vi "S4GUI.vi"(7 "Tab ObsEng":enum32{"Obs", "CCD modes", "Eng"}(tab)) -> ()   [LabVIEW 2018] (continued)
            n3222 = call-dynamic "Write ObsType.vi"("error in (no error)"=w7236, "ObsType"=w7222, "Interface in"=w7230) -> ("error out"=w7235:errorcluster, "Interface out"=w7229:refnum<class "Interface.lvclass">)  [unwired: 7 in]
            n3223 = call-dynamic "Write Object.vi"("error in (no error)"=w7235, "Object"=w7221, "Interface in"=w7229) -> ("error out"=w7234:errorcluster, "Interface out"=w7228:refnum<class "Interface.lvclass">)  [unwired: 7 in]
            n3224 = call-dynamic "Write Comments.vi"("error in (no error)"=w7234, "Comments"=w7223, "Interface in"=w7228) -> ("error out"=w7215:errorcluster, "Interface out"=w7214:refnum<class "Interface.lvclass">)  [unwired: 7 in]
            n3225 = call-dynamic "Write Observer.vi"("error in (no error)"=w7215, "Observer"=w7220, "Interface in"=w7214) -> ("error out"=w7216:errorcluster, "Interface out"=w7217:refnum<class "Interface.lvclass">)  [unwired: 7 in]
            n3226 = call-dynamic "Write Interface.vi"("error in (no error)"=w7216, "Interface.lvclass"=w7217, "Channel in"=w7231) -> ("error out"=w7212:errorcluster, "Channel out"=w7213:refnum<class "Channel.lvclass">)  [unwired: 7 in]
            n3227 = disable-structure shown="Enabled" {
              disable-tunnel: w7213 -> [w7248 w7253]
              disable-tunnel: w7212 -> [w7247 w7252]
              disable-tunnel: [w7245 w7253] -> w7211
              disable-tunnel: [w7242 w7252] -> w7210
              frame Disabled {
                n3228 = call-dynamic "Read State Machine.vi"("error in (no error)"=w7247, "Device in"=w7248) -> ("error out"=w7251:errorcluster, "State Machine.lvclass"=w7244:refnum<class "State Machine.lvclass">, "Device out"=w7246:refnum<class "Channel.lvclass">)  [unwired: 7 in]
                n3229 = call "Next State.vi"("error in (no error)"=w7251, "New_State"=12, "State Machine in"=w7244) -> ("error out"=w7250:errorcluster, "State Machine out"=w7243:refnum<class "State Machine.lvclass">)  [unwired: 7 in]
                n3230 = call-dynamic "Write State Machine.vi"("error in (no error)"=w7250, "State Machine.lvclass"=w7243, "Device in"=w7246) -> ("error out"=w7242:errorcluster, "Device out"=w7245:refnum<class "Channel.lvclass">)  [unwired: 7 in]
              }
              frame Enabled {
              }
            }
            n3231 = call-dynamic "Write Channel.vi"("error in (no error)"=w7210, "Channel.lvclass"=w7211, "Acquisition in"=w7226) -> ("error out"=w7224:errorcluster, "Acquisition out"=w7225:refnum<class "Acquisition.lvclass">)  [unwired: 7 in]
            n3232 = call-dynamic "Write AcquisitionC.vi"("error in (no error)"=w7224, "Acquisition.lvclass"=w7225, "S4ACS_GUI in"=w7227) -> ("error out"=w7238:errorcluster, "S4ACS_GUI out"=w7239:refnum<class "S4GUI.lvclass">)  [unwired: 7 in]
          }
          frame #3 {
            # "object"
            # "suffix"
            # "obsType"
            n3233 = call-dynamic "Read AcquisitionD.vi"("error in (no error)"=w7289, "S4ACS_GUI in"=w7290) -> ("error out"=w7282:errorcluster, "Acquisition.lvclass"=w7281:refnum<class "Acquisition.lvclass">, "S4ACS_GUI out"=w7276:refnum<class "S4GUI.lvclass">)  [unwired: 7 in]
            n3234 = call-dynamic "Read Channel.vi"("error in (no error)"=w7282, "Acquisition in"=w7281) -> ("error out"=w7255:errorcluster, "Channel.lvclass"=w7257:refnum<class "Channel.lvclass">, "Acquisition out"=w7275:refnum<class "Acquisition.lvclass">)  [unwired: 7 in]
            n3235 = local read "Filter4"() -> (w7258:u8)
            n3236 = call-dynamic "Write Filter.vi"("error in (no error)"=w7255, "Filter"=w7258, "Channel in"=w7257) -> ("error out"=w7254:errorcluster, "Channel out"=w7256:refnum<class "Channel.lvclass">)  [unwired: 7 in]
            n3237 = call-dynamic "Read Interface.vi"("error in (no error)"=w7254, "Channel in"=w7256) -> ("error out"=w7267:errorcluster, "Interface.lvclass"=w7268:refnum<class "Interface.lvclass">, "Channel out"=w7280:refnum<class "Channel.lvclass">)  [unwired: 7 in]
            n3238 = call-dynamic "Write Suffix.vi"("error in (no error)"=w7267, "Suffix"=w7286, "Interface in"=w7268) -> ("error out"=w7285:errorcluster, "Interface out"=w7279:refnum<class "Interface.lvclass">)  [unwired: 7 in]
            n3239 = call-dynamic "Write ObsType.vi"("error in (no error)"=w7285, "ObsType"=w7271, "Interface in"=w7279) -> ("error out"=w7284:errorcluster, "Interface out"=w7278:refnum<class "Interface.lvclass">)  [unwired: 7 in]
            n3240 = call-dynamic "Write Object.vi"("error in (no error)"=w7284, "Object"=w7270, "Interface in"=w7278) -> ("error out"=w7283:errorcluster, "Interface out"=w7277:refnum<class "Interface.lvclass">)  [unwired: 7 in]
            n3241 = call-dynamic "Write Comments.vi"("error in (no error)"=w7283, "Comments"=w7272, "Interface in"=w7277) -> ("error out"=w7266:errorcluster, "Interface out"=w7265:refnum<class "Interface.lvclass">)  [unwired: 7 in]
            n3242 = call-dynamic "Write Observer.vi"("error in (no error)"=w7266, "Observer"=w7269, "Interface in"=w7265) -> ("error out"=w7264:errorcluster, "Interface out"=w7263:refnum<class "Interface.lvclass">)  [unwired: 7 in]
            n3243 = call-dynamic "Write Interface.vi"("error in (no error)"=w7264, "Interface.lvclass"=w7263, "Channel in"=w7280) -> ("error out"=w7260:errorcluster, "Channel out"=w7262:refnum<class "Channel.lvclass">)  [unwired: 7 in]
            n3244 = disable-structure shown="Enabled" {
              disable-tunnel: w7262 -> [w7297 w7302]
              disable-tunnel: [w7295 w7302] -> w7261
              disable-tunnel: w7260 -> [w7294 w7301]
              disable-tunnel: [w7293 w7301] -> w7259
              frame Disabled {
                n3245 = call-dynamic "Read State Machine.vi"("error in (no error)"=w7294, "Device in"=w7297) -> ("error out"=w7300:errorcluster, "State Machine.lvclass"=w7292:refnum<class "State Machine.lvclass">, "Device out"=w7296:refnum<class "Channel.lvclass">)  [unwired: 7 in]
                n3246 = call "Next State.vi"("error in (no error)"=w7300, "New_State"=12, "State Machine in"=w7292) -> ("error out"=w7299:errorcluster, "State Machine out"=w7291:refnum<class "State Machine.lvclass">)  [unwired: 7 in]
                n3247 = call-dynamic "Write State Machine.vi"("error in (no error)"=w7299, "State Machine.lvclass"=w7291, "Device in"=w7296) -> ("error out"=w7293:errorcluster, "Device out"=w7295:refnum<class "Channel.lvclass">)  [unwired: 7 in]
              }
              frame Enabled {
              }
            }
            n3248 = call-dynamic "Write Channel.vi"("error in (no error)"=w7259, "Channel.lvclass"=w7261, "Acquisition in"=w7275) -> ("error out"=w7273:errorcluster, "Acquisition out"=w7274:refnum<class "Acquisition.lvclass">)  [unwired: 7 in]
            n3249 = call-dynamic "Write AcquisitionD.vi"("error in (no error)"=w7273, "Acquisition.lvclass"=w7274, "S4ACS_GUI in"=w7276) -> ("error out"=w7287:errorcluster, "S4ACS_GUI out"=w7288:refnum<class "S4GUI.lvclass">)  [unwired: 7 in]
          }
        }
      }
      event "Observer": Value Change {
        n3250 = event-data() -> ("NewVal"=w7303:string)  [unwired: 1 in, 5 out]
        n3251 = disable-structure shown="Disabled" {
          disable-tunnel: w7306 -> [w7321 w7322]
          disable-tunnel: w7303 -> [w7320 _]
          disable-tunnel: [w7319 w7322] -> w7305
          frame Disabled {
            n3252 = String Length(string=w7320) -> (length=w7318:i32)
            n3253 = Equal To 0?(x=w7318) -> (x = 0?=w7317:bool)
            n3254 = Select(t=u32 16777216, s=w7317, f=u32 16777225) -> (s? t:f=w7315:u32)
            n3255 = property on="Observer" class="Str"(error in=w7321, "Text.BGColor"=w7315) -> (error out=w7319:errorcluster)  [unwired: 1 in, 1 out]
          }
          frame Enabled {
            # "Não se usa mais o texto de fundo\ndo controle \"Observer\""
          }
        }
        n3256 = case shown="False" FALSE {
          tunnel: w7313 -> [w7331 w7529]
          tunnel: w7312 -> [w7330 _]
          tunnel: w7311 -> [w7329 _]
          tunnel: w7310 -> [w7328 _]
          tunnel: w7303 -> [w7327 _]
          tunnel: w7309 -> [w7326 _]
          tunnel: [w7325 w7529] -> w7308
          tunnel: [w7324 w7528] -> w7307
          tunnel: w7305 -> [w7323 w7528]
          frame False {
            n3257 = stacked-sequence {
              seq-local: [w7353 _ _ _] -> [_ w7417 _ _]
              seq-local: [w7352 _ _ _] -> [_ w7416 _ _]
              seq-local: [_ w7415 _ _] -> [_ _ w7466 _]
              seq-local: [_ w7414 _ _] -> [_ _ w7465 _]
              seq-local: [_ _ w7464 _] -> [_ _ _ w7515]
              seq-local: [_ _ w7463 _] -> [_ _ _ w7514]
              tunnel: w7323 -> [w7365 _ _ _]
              tunnel: w7331 -> [w7364 _ _ _]
              tunnel: [_ _ _ w7513] -> w7325
              tunnel: [_ _ _ w7512] -> w7324
              tunnel: w7329 -> [w7351 w7413 w7462 w7511]
              tunnel: w7328 -> [w7350 w7412 w7448 w7497]
              tunnel: w7326 -> [w7349 w7398 w7447 w7496]
              tunnel: w7330 -> [w7348 w7397 w7446 w7495]
              tunnel: w7327 -> [w7347 w7396 w7445 w7494]
              frame #0 {
                # "observer"
                # "comment"
                # "object"
                # "suffix"
                # "obsType"
                n3258 = call-dynamic "Read AcquisitionA.vi"("error in (no error)"=w7365, "S4ACS_GUI in"=w7364) -> ("error out"=w7363:errorcluster, "Acquisition.lvclass"=w7362:refnum<class "Acquisition.lvclass">, "S4ACS_GUI out"=w7357:refnum<class "S4GUI.lvclass">)  [unwired: 7 in]
                n3259 = call-dynamic "Read Channel.vi"("error in (no error)"=w7363, "Acquisition in"=w7362) -> ("error out"=w7333:errorcluster, "Channel.lvclass"=w7336:refnum<class "Channel.lvclass">, "Acquisition out"=w7356:refnum<class "Acquisition.lvclass">)  [unwired: 7 in]
                n3260 = local read "Filter1"() -> (w7334:u8)
                n3261 = call-dynamic "Write Filter.vi"("error in (no error)"=w7333, "Filter"=w7334, "Channel in"=w7336) -> ("error out"=w7332:errorcluster, "Channel out"=w7335:refnum<class "Channel.lvclass">)  [unwired: 7 in]
                n3262 = call-dynamic "Read Interface.vi"("error in (no error)"=w7332, "Channel in"=w7335) -> ("error out"=w7343:errorcluster, "Interface.lvclass"=w7344:refnum<class "Interface.lvclass">, "Channel out"=w7361:refnum<class "Channel.lvclass">)  [unwired: 7 in]
                n3263 = call-dynamic "Write Suffix.vi"("error in (no error)"=w7343, "Suffix"=w7351, "Interface in"=w7344) -> ("error out"=w7368:errorcluster, "Interface out"=w7360:refnum<class "Interface.lvclass">)  [unwired: 7 in]
                n3264 = call-dynamic "Write ObsType.vi"("error in (no error)"=w7368, "ObsType"=w7349, "Interface in"=w7360) -> ("error out"=w7367:errorcluster, "Interface out"=w7359:refnum<class "Interface.lvclass">)  [unwired: 7 in]
                n3265 = call-dynamic "Write Object.vi"("error in (no error)"=w7367, "Object"=w7348, "Interface in"=w7359) -> ("error out"=w7366:errorcluster, "Interface out"=w7358:refnum<class "Interface.lvclass">)  [unwired: 7 in]
                n3266 = call-dynamic "Write Comments.vi"("error in (no error)"=w7366, "Comments"=w7350, "Interface in"=w7358) -> ("error out"=w7346:errorcluster, "Interface out"=w7345:refnum<class "Interface.lvclass">)  [unwired: 7 in]
                n3267 = call-dynamic "Write Observer.vi"("error in (no error)"=w7346, "Observer"=w7347, "Interface in"=w7345) -> ("error out"=w7341:errorcluster, "Interface out"=w7342:refnum<class "Interface.lvclass">)  [unwired: 7 in]
                n3268 = call-dynamic "Write Interface.vi"("error in (no error)"=w7341, "Interface.lvclass"=w7342, "Channel in"=w7361) -> ("error out"=w7338:errorcluster, "Channel out"=w7340:refnum<class "Channel.lvclass">)  [unwired: 7 in]
                n3269 = disable-structure shown="Enabled" {
                  disable-tunnel: w7340 -> [w7378 w7380]
                  disable-tunnel: [w7376 w7380] -> w7339
                  disable-tunnel: w7338 -> [w7375 w7379]
                  disable-tunnel: [w7370 w7379] -> w7337
                  frame Disabled {
                    n3270 = call-dynamic "Read State Machine.vi"("error in (no error)"=w7375, "Device in"=w7378) -> ("error out"=w7374:errorcluster, "State Machine.lvclass"=w7372:refnum<class "State Machine.lvclass">, "Device out"=w7377:refnum<class "Channel.lvclass">)  [unwired: 7 in]
                    n3271 = call "Next State.vi"("error in (no error)"=w7374, "New_State"=12, "State Machine in"=w7372) -> ("error out"=w7373:errorcluster, "State Machine out"=w7371:refnum<class "State Machine.lvclass">)  [unwired: 7 in]
                    n3272 = call-dynamic "Write State Machine.vi"("error in (no error)"=w7373, "State Machine.lvclass"=w7371, "Device in"=w7377) -> ("error out"=w7370:errorcluster, "Device out"=w7376:refnum<class "Channel.lvclass">)  [unwired: 7 in]
                  }
                  frame Enabled {
                  }
                }
                n3273 = call-dynamic "Write Channel.vi"("error in (no error)"=w7337, "Channel.lvclass"=w7339, "Acquisition in"=w7356) -> ("error out"=w7354:errorcluster, "Acquisition out"=w7355:refnum<class "Acquisition.lvclass">)  [unwired: 7 in]
                n3274 = call-dynamic "Write AcquisitionA.vi"("error in (no error)"=w7354, "Acquisition.lvclass"=w7355, "S4ACS_GUI in"=w7357) -> ("error out"=w7352:errorcluster, "S4ACS_GUI out"=w7353:refnum<class "S4GUI.lvclass">)  [unwired: 7 in]
              }
              frame #1 {
                # "object"
                # "suffix"
                # "obsType"
                n3275 = call "Read AcquisitionB.vi"("error in (no error)"=w7416, "S4ACS_GUI in"=w7417) -> ("error out"=w7402:errorcluster, "Acquisition.lvclass"=w7403:refnum<class "Acquisition.lvclass">, "S4ACS_GUI out"=w7408:refnum<class "S4GUI.lvclass">)  [unwired: 7 in]
                n3276 = call-dynamic "Read Channel.vi"("error in (no error)"=w7402, "Acquisition in"=w7403) -> ("error out"=w7382:errorcluster, "Channel.lvclass"=w7384:refnum<class "Channel.lvclass">, "Acquisition out"=w7409:refnum<class "Acquisition.lvclass">)  [unwired: 7 in]
                n3277 = local read "Filter2"() -> (w7385:u8)
                n3278 = call-dynamic "Write Filter.vi"("error in (no error)"=w7382, "Filter"=w7385, "Channel in"=w7384) -> ("error out"=w7381:errorcluster, "Channel out"=w7383:refnum<class "Channel.lvclass">)  [unwired: 7 in]
                n3279 = call-dynamic "Read Interface.vi"("error in (no error)"=w7381, "Channel in"=w7383) -> ("error out"=w7390:errorcluster, "Interface.lvclass"=w7391:refnum<class "Interface.lvclass">, "Channel out"=w7404:refnum<class "Channel.lvclass">)  [unwired: 7 in]
                n3280 = call-dynamic "Write Suffix.vi"("error in (no error)"=w7390, "Suffix"=w7413, "Interface in"=w7391) -> ("error out"=w7399:errorcluster, "Interface out"=w7405:refnum<class "Interface.lvclass">)  [unwired: 7 in]
                n3281 = call-dynamic "Write ObsType.vi"("error in (no error)"=w7399, "ObsType"=w7398, "Interface in"=w7405) -> ("error out"=w7400:errorcluster, "Interface out"=w7406:refnum<class "Interface.lvclass">)  [unwired: 7 in]
                n3282 = call-dynamic "Write Object.vi"("error in (no error)"=w7400, "Object"=w7397, "Interface in"=w7406) -> ("error out"=w7401:errorcluster, "Interface out"=w7407:refnum<class "Interface.lvclass">)  [unwired: 7 in]
                n3283 = call-dynamic "Write Comments.vi"("error in (no error)"=w7401, "Comments"=w7412, "Interface in"=w7407) -> ("error out"=w7393:errorcluster, "Interface out"=w7392:refnum<class "Interface.lvclass">)  [unwired: 7 in]
                n3284 = call-dynamic "Write Observer.vi"("error in (no error)"=w7393, "Observer"=w7396, "Interface in"=w7392) -> ("error out"=w7394:errorcluster, "Interface out"=w7395:refnum<class "Interface.lvclass">)  [unwired: 7 in]
                n3285 = call-dynamic "Write Interface.vi"("error in (no error)"=w7394, "Interface.lvclass"=w7395, "Channel in"=w7404) -> ("error out"=w7388:errorcluster, "Channel out"=w7389:refnum<class "Channel.lvclass">)  [unwired: 7 in]
                n3286 = disable-structure shown="Enabled" {
                  disable-tunnel: w7389 -> [w7422 w7429]
                  disable-tunnel: w7388 -> [w7421 w7428]
                  disable-tunnel: [w7419 w7429] -> w7387
                  disable-tunnel: [w7418 w7428] -> w7386
                  frame Disabled {
                    n3287 = call-dynamic "Read State Machine.vi"("error in (no error)"=w7421, "Device in"=w7422) -> ("error out"=w7427:errorcluster, "State Machine.lvclass"=w7425:refnum<class "State Machine.lvclass">, "Device out"=w7420:refnum<class "Channel.lvclass">)  [unwired: 7 in]
                    n3288 = call "Next State.vi"("error in (no error)"=w7427, "New_State"=12, "State Machine in"=w7425) -> ("error out"=w7426:errorcluster, "State Machine out"=w7424:refnum<class "State Machine.lvclass">)  [unwired: 7 in]
                    n3289 = call-dynamic "Write State Machine.vi"("error in (no error)"=w7426, "State Machine.lvclass"=w7424, "Device in"=w7420) -> ("error out"=w7418:errorcluster, "Device out"=w7419:refnum<class "Channel.lvclass">)  [unwired: 7 in]
                  }
                  frame Enabled {
                  }
                }
                n3290 = call-dynamic "Write Channel.vi"("error in (no error)"=w7386, "Channel.lvclass"=w7387, "Acquisition in"=w7409) -> ("error out"=w7411:errorcluster, "Acquisition out"=w7410:refnum<class "Acquisition.lvclass">)  [unwired: 7 in]
                n3291 = call "Write AcquisitionB.vi"("error in (no error)"=w7411, "Acquisition.lvclass"=w7410, "S4ACS_GUI in"=w7408) -> ("error out"=w7414:errorcluster, "S4ACS_GUI out"=w7415:refnum<class "S4GUI.lvclass">)  [unwired: 7 in]
              }
              frame #2 {
                # "object"
                # "suffix"
                # "obsType"
                n3292 = call-dynamic "Read AcquisitionC.vi"("error in (no error)"=w7465, "S4ACS_GUI in"=w7466) -> ("error out"=w7458:errorcluster, "Acquisition.lvclass"=w7457:refnum<class "Acquisition.lvclass">, "S4ACS_GUI out"=w7452:refnum<class "S4GUI.lvclass">)  [unwired: 7 in]
                n3293 = call-dynamic "Read Channel.vi"("error in (no error)"=w7458, "Acquisition in"=w7457) -> ("error out"=w7431:errorcluster, "Channel.lvclass"=w7433:refnum<class "Channel.lvclass">, "Acquisition out"=w7451:refnum<class "Acquisition.lvclass">)  [unwired: 7 in]
                n3294 = local read "Filter3"() -> (w7434:u8)
                n3295 = call-dynamic "Write Filter.vi"("error in (no error)"=w7431, "Filter"=w7434, "Channel in"=w7433) -> ("error out"=w7430:errorcluster, "Channel out"=w7432:refnum<class "Channel.lvclass">)  [unwired: 7 in]
                n3296 = call-dynamic "Read Interface.vi"("error in (no error)"=w7430, "Channel in"=w7432) -> ("error out"=w7443:errorcluster, "Interface.lvclass"=w7444:refnum<class "Interface.lvclass">, "Channel out"=w7456:refnum<class "Channel.lvclass">)  [unwired: 7 in]
                n3297 = call-dynamic "Write Suffix.vi"("error in (no error)"=w7443, "Suffix"=w7462, "Interface in"=w7444) -> ("error out"=w7461:errorcluster, "Interface out"=w7455:refnum<class "Interface.lvclass">)  [unwired: 7 in]
                n3298 = call-dynamic "Write ObsType.vi"("error in (no error)"=w7461, "ObsType"=w7447, "Interface in"=w7455) -> ("error out"=w7460:errorcluster, "Interface out"=w7454:refnum<class "Interface.lvclass">)  [unwired: 7 in]
                n3299 = call-dynamic "Write Object.vi"("error in (no error)"=w7460, "Object"=w7446, "Interface in"=w7454) -> ("error out"=w7459:errorcluster, "Interface out"=w7453:refnum<class "Interface.lvclass">)  [unwired: 7 in]
                n3300 = call-dynamic "Write Comments.vi"("error in (no error)"=w7459, "Comments"=w7448, "Interface in"=w7453) -> ("error out"=w7440:errorcluster, "Interface out"=w7439:refnum<class "Interface.lvclass">)  [unwired: 7 in]
                n3301 = call-dynamic "Write Observer.vi"("error in (no error)"=w7440, "Observer"=w7445, "Interface in"=w7439) -> ("error out"=w7441:errorcluster, "Interface out"=w7442:refnum<class "Interface.lvclass">)  [unwired: 7 in]
                n3302 = call-dynamic "Write Interface.vi"("error in (no error)"=w7441, "Interface.lvclass"=w7442, "Channel in"=w7456) -> ("error out"=w7437:errorcluster, "Channel out"=w7438:refnum<class "Channel.lvclass">)  [unwired: 7 in]
                n3303 = disable-structure shown="Enabled" {
                  disable-tunnel: w7438 -> [w7473 w7478]
                  disable-tunnel: w7437 -> [w7472 w7477]
                  disable-tunnel: [w7470 w7478] -> w7436
                  disable-tunnel: [w7467 w7477] -> w7435
                  frame Disabled {
                    n3304 = call-dynamic "Read State Machine.vi"("error in (no error)"=w7472, "Device in"=w7473) -> ("error out"=w7476:errorcluster, "State Machine.lvclass"=w7469:refnum<class "State Machine.lvclass">, "Device out"=w7471:refnum<class "Channel.lvclass">)  [unwired: 7 in]
                    n3305 = call "Next State.vi"("error in (no error)"=w7476, "New_State"=12, "State Machine in"=w7469) -> ("error out"=w7475:errorcluster, "State Machine out"=w7468:refnum<class "State Machine.lvclass">)  [unwired: 7 in]
                    n3306 = call-dynamic "Write State Machine.vi"("error in (no error)"=w7475, "State Machine.lvclass"=w7468, "Device in"=w7471) -> ("error out"=w7467:errorcluster, "Device out"=w7470:refnum<class "Channel.lvclass">)  [unwired: 7 in]
                  }
                  frame Enabled {
                  }
                }
                n3307 = call-dynamic "Write Channel.vi"("error in (no error)"=w7435, "Channel.lvclass"=w7436, "Acquisition in"=w7451) -> ("error out"=w7449:errorcluster, "Acquisition out"=w7450:refnum<class "Acquisition.lvclass">)  [unwired: 7 in]
                n3308 = call-dynamic "Write AcquisitionC.vi"("error in (no error)"=w7449, "Acquisition.lvclass"=w7450, "S4ACS_GUI in"=w7452) -> ("error out"=w7463:errorcluster, "S4ACS_GUI out"=w7464:refnum<class "S4GUI.lvclass">)  [unwired: 7 in]
              }
              frame #3 {
                # "object"
                # "suffix"
                # "obsType"
                n3309 = call-dynamic "Read AcquisitionD.vi"("error in (no error)"=w7514, "S4ACS_GUI in"=w7515) -> ("error out"=w7507:errorcluster, "Acquisition.lvclass"=w7506:refnum<class "Acquisition.lvclass">, "S4ACS_GUI out"=w7501:refnum<class "S4GUI.lvclass">)  [unwired: 7 in]
                n3310 = call-dynamic "Read Channel.vi"("error in (no error)"=w7507, "Acquisition in"=w7506) -> ("error out"=w7480:errorcluster, "Channel.lvclass"=w7482:refnum<class "Channel.lvclass">, "Acquisition out"=w7500:refnum<class "Acquisition.lvclass">)  [unwired: 7 in]
                n3311 = local read "Filter4"() -> (w7483:u8)
                n3312 = call-dynamic "Write Filter.vi"("error in (no error)"=w7480, "Filter"=w7483, "Channel in"=w7482) -> ("error out"=w7479:errorcluster, "Channel out"=w7481:refnum<class "Channel.lvclass">)  [unwired: 7 in]
                n3313 = call-dynamic "Read Interface.vi"("error in (no error)"=w7479, "Channel in"=w7481) -> ("error out"=w7492:errorcluster, "Interface.lvclass"=w7493:refnum<class "Interface.lvclass">, "Channel out"=w7505:refnum<class "Channel.lvclass">)  [unwired: 7 in]
                n3314 = call-dynamic "Write Suffix.vi"("error in (no error)"=w7492, "Suffix"=w7511, "Interface in"=w7493) -> ("error out"=w7510:errorcluster, "Interface out"=w7504:refnum<class "Interface.lvclass">)  [unwired: 7 in]
                n3315 = call-dynamic "Write ObsType.vi"("error in (no error)"=w7510, "ObsType"=w7496, "Interface in"=w7504) -> ("error out"=w7509:errorcluster, "Interface out"=w7503:refnum<class "Interface.lvclass">)  [unwired: 7 in]
                n3316 = call-dynamic "Write Object.vi"("error in (no error)"=w7509, "Object"=w7495, "Interface in"=w7503) -> ("error out"=w7508:errorcluster, "Interface out"=w7502:refnum<class "Interface.lvclass">)  [unwired: 7 in]
                n3317 = call-dynamic "Write Comments.vi"("error in (no error)"=w7508, "Comments"=w7497, "Interface in"=w7502) -> ("error out"=w7491:errorcluster, "Interface out"=w7490:refnum<class "Interface.lvclass">)  [unwired: 7 in]
                n3318 = call-dynamic "Write Observer.vi"("error in (no error)"=w7491, "Observer"=w7494, "Interface in"=w7490) -> ("error out"=w7489:errorcluster, "Interface out"=w7488:refnum<class "Interface.lvclass">)  [unwired: 7 in]
                n3319 = call-dynamic "Write Interface.vi"("error in (no error)"=w7489, "Interface.lvclass"=w7488, "Channel in"=w7505) -> ("error out"=w7485:errorcluster, "Channel out"=w7487:refnum<class "Channel.lvclass">)  [unwired: 7 in]
                n3320 = disable-structure shown="Enabled" {
                  disable-tunnel: w7487 -> [w7522 w7527]
                  disable-tunnel: [w7520 w7527] -> w7486
                  disable-tunnel: w7485 -> [w7519 w7526]
                  disable-tunnel: [w7518 w7526] -> w7484
                  frame Disabled {
                    n3321 = call-dynamic "Read State Machine.vi"("error in (no error)"=w7519, "Device in"=w7522) -> ("error out"=w7525:errorcluster, "State Machine.lvclass"=w7517:refnum<class "State Machine.lvclass">, "Device out"=w7521:refnum<class "Channel.lvclass">)  [unwired: 7 in]
                    n3322 = call "Next State.vi"("error in (no error)"=w7525, "New_State"=12, "State Machine in"=w7517) -> ("error out"=w7524:errorcluster, "State Machine out"=w7516:refnum<class "State Machine.lvclass">)  [unwired: 7 in]
                    n3323 = call-dynamic "Write State Machine.vi"("error in (no error)"=w7524, "State Machine.lvclass"=w7516, "Device in"=w7521) -> ("error out"=w7518:errorcluster, "Device out"=w7520:refnum<class "Channel.lvclass">)  [unwired: 7 in]
                  }
                  frame Enabled {
                  }
                }
                n3324 = call-dynamic "Write Channel.vi"("error in (no error)"=w7484, "Channel.lvclass"=w7486, "Acquisition in"=w7500) -> ("error out"=w7498:errorcluster, "Acquisition out"=w7499:refnum<class "Acquisition.lvclass">)  [unwired: 7 in]
                n3325 = call-dynamic "Write AcquisitionD.vi"("error in (no error)"=w7498, "Acquisition.lvclass"=w7499, "S4ACS_GUI in"=w7501) -> ("error out"=w7512:errorcluster, "S4ACS_GUI out"=w7513:refnum<class "S4GUI.lvclass">)  [unwired: 7 in]
              }
            }
          }
          frame True {
          }
        }
      }
      event "Observer": Mouse Enter {
        n3326 = event-data() -> ()  [unwired: 1 in, 4 out]
        n3327 = disable-structure shown="Disabled" {
          disable-tunnel: [w7535 w7538] -> w7531
          disable-tunnel: w7530 -> [w7533 w7538]
          frame Disabled {
            n3328 = property on="Observer" class="Str"() -> ("Value"=w7534:string)  [unwired: 2 in, 2 out]
            n3329 = String Length(string=w7534) -> (length=w7537:i32)
            n3330 = Equal To 0?(x=w7537) -> (x = 0?=w7536:bool)
            n3331 = property on="Observer" class="Str"(error in=w7533, "Caption.Visible"=w7536) -> (error out=w7535:errorcluster)  [unwired: 1 in, 1 out]
          }
          frame Enabled {
            # "Não se usa mais o texto de fundo\ndo controle \"Observer\""
          }
        }
      }
      event "Filter1", "Filter2", "Filter3", "Filter4": Value Change {
        n3332 = event-data() -> ()  [unwired: 1 in, 6 out]
        n3333 = stacked-sequence {
          seq-local: [w7569 _ _ _] -> [_ w7633 _ _]
          seq-local: [w7568 _ _ _] -> [_ w7632 _ _]
          seq-local: [_ w7631 _ _] -> [_ _ w7682 _]
          seq-local: [_ w7630 _ _] -> [_ _ w7681 _]
          seq-local: [_ _ w7680 _] -> [_ _ _ w7731]
          seq-local: [_ _ w7679 _] -> [_ _ _ w7730]
          tunnel: w7546 -> [w7581 _ _ _]
          tunnel: w7547 -> [w7580 _ _ _]
          tunnel: [_ _ _ w7729] -> w7540
          tunnel: [_ _ _ w7728] -> w7539
          tunnel: w7544 -> [w7567 w7629 w7678 w7727]
          tunnel: w7543 -> [w7566 w7628 w7664 w7713]
          tunnel: w7541 -> [w7565 w7614 w7663 w7712]
          tunnel: w7545 -> [w7564 w7613 w7662 w7711]
          tunnel: w7542 -> [w7563 w7612 w7661 w7710]
          frame #0 {
            # "observer"
            # "comment"
            # "object"
            # "suffix"
            # "obsType"
            n3334 = call-dynamic "Read AcquisitionA.vi"("error in (no error)"=w7581, "S4ACS_GUI in"=w7580) -> ("error out"=w7579:errorcluster, "Acquisition.lvclass"=w7578:refnum<class "Acquisition.lvclass">, "S4ACS_GUI out"=w7573:refnum<class "S4GUI.lvclass">)  [unwired: 7 in]
            n3335 = call-dynamic "Read Channel.vi"("error in (no error)"=w7579, "Acquisition in"=w7578) -> ("error out"=w7549:errorcluster, "Channel.lvclass"=w7552:refnum<class "Channel.lvclass">, "Acquisition out"=w7572:refnum<class "Acquisition.lvclass">)  [unwired: 7 in]
            n3336 = local read "Filter1"() -> (w7550:u8)
            n3337 = call-dynamic "Write Filter.vi"("error in (no error)"=w7549, "Filter"=w7550, "Channel in"=w7552) -> ("error out"=w7548:errorcluster, "Channel out"=w7551:refnum<class "Channel.lvclass">)  [unwired: 7 in]
            n3338 = call-dynamic "Read Interface.vi"("error in (no error)"=w7548, "Channel in"=w7551) -> ("error out"=w7559:errorcluster, "Interface.lvclass"=w7560:refnum<class "Interface.lvclass">, "Channel out"=w7577:refnum<class "Channel.lvclass">)  [unwired: 7 in]
            n3339 = call-dynamic "Write Suffix.vi"("error in (no error)"=w7559, "Suffix"=w7567, "Interface in"=w7560) -> ("error out"=w7584:errorcluster, "Interface out"=w7576:refnum<class "Interface.lvclass">)  [unwired: 7 in]
            n3340 = call-dynamic "Write ObsType.vi"("error in (no error)"=w7584, "ObsType"=w7565, "Interface in"=w7576) -> ("error out"=w7583:errorcluster, "Interface out"=w7575:refnum<class "Interface.lvclass">)  [unwired: 7 in]
            n3341 = call-dynamic "Write Object.vi"("error in (no error)"=w7583, "Object"=w7564, "Interface in"=w7575) -> ("error out"=w7582:errorcluster, "Interface out"=w7574:refnum<class "Interface.lvclass">)  [unwired: 7 in]
            n3342 = call-dynamic "Write Comments.vi"("error in (no error)"=w7582, "Comments"=w7566, "Interface in"=w7574) -> ("error out"=w7562:errorcluster, "Interface out"=w7561:refnum<class "Interface.lvclass">)  [unwired: 7 in]
            n3343 = call-dynamic "Write Observer.vi"("error in (no error)"=w7562, "Observer"=w7563, "Interface in"=w7561) -> ("error out"=w7557:errorcluster, "Interface out"=w7558:refnum<class "Interface.lvclass">)  [unwired: 7 in]
            n3344 = call-dynamic "Write Interface.vi"("error in (no error)"=w7557, "Interface.lvclass"=w7558, "Channel in"=w7577) -> ("error out"=w7554:errorcluster, "Channel out"=w7556:refnum<class "Channel.lvclass">)  [unwired: 7 in]
            n3345 = disable-structure shown="Enabled" {
              disable-tunnel: w7556 -> [w7594 w7596]
              disable-tunnel: [w7592 w7596] -> w7555
              disable-tunnel: w7554 -> [w7591 w7595]
              disable-tunnel: [w7586 w7595] -> w7553
              frame Disabled {
                n3346 = call-dynamic "Read State Machine.vi"("error in (no error)"=w7591, "Device in"=w7594) -> ("error out"=w7590:errorcluster, "State Machine.lvclass"=w7588:refnum<class "State Machine.lvclass">, "Device out"=w7593:refnum<class "Channel.lvclass">)  [unwired: 7 in]
                n3347 = call "Next State.vi"("error in (no error)"=w7590, "New_State"=12, "State Machine in"=w7588) -> ("error out"=w7589:errorcluster, "State Machine out"=w7587:refnum<class "State Machine.lvclass">)  [unwired: 7 in]
                n3348 = call-dynamic "Write State Machine.vi"("error in (no error)"=w7589, "State Machine.lvclass"=w7587, "Device in"=w7593) -> ("error out"=w7586:errorcluster, "Device out"=w7592:refnum<class "Channel.lvclass">)  [unwired: 7 in]
              }
              frame Enabled {
              }
            }
            n3349 = call-dynamic "Write Channel.vi"("error in (no error)"=w7553, "Channel.lvclass"=w7555, "Acquisition in"=w7572) -> ("error out"=w7570:errorcluster, "Acquisition out"=w7571:refnum<class "Acquisition.lvclass">)  [unwired: 7 in]
            n3350 = call-dynamic "Write AcquisitionA.vi"("error in (no error)"=w7570, "Acquisition.lvclass"=w7571, "S4ACS_GUI in"=w7573) -> ("error out"=w7568:errorcluster, "S4ACS_GUI out"=w7569:refnum<class "S4GUI.lvclass">)  [unwired: 7 in]
          }
          frame #1 {
            # "object"
            # "suffix"
            # "obsType"
            n3351 = call "Read AcquisitionB.vi"("error in (no error)"=w7632, "S4ACS_GUI in"=w7633) -> ("error out"=w7618:errorcluster, "Acquisition.lvclass"=w7619:refnum<class "Acquisition.lvclass">, "S4ACS_GUI out"=w7624:refnum<class "S4GUI.lvclass">)  [unwired: 7 in]
            n3352 = call-dynamic "Read Channel.vi"("error in (no error)"=w7618, "Acquisition in"=w7619) -> ("error out"=w7598:errorcluster, "Channel.lvclass"=w7600:refnum<class "Channel.lvclass">, "Acquisition out"=w7625:refnum<class "Acquisition.lvclass">)  [unwired: 7 in]
            n3353 = local read "Filter2"() -> (w7601:u8)
            n3354 = call-dynamic "Write Filter.vi"("error in (no error)"=w7598, "Filter"=w7601, "Channel in"=w7600) -> ("error out"=w7597:errorcluster, "Channel out"=w7599:refnum<class "Channel.lvclass">)  [unwired: 7 in]
            n3355 = call-dynamic "Read Interface.vi"("error in (no error)"=w7597, "Channel in"=w7599) -> ("error out"=w7606:errorcluster, "Interface.lvclass"=w7607:refnum<class "Interface.lvclass">, "Channel out"=w7620:refnum<class "Channel.lvclass">)  [unwired: 7 in]
            n3356 = call-dynamic "Write Suffix.vi"("error in (no error)"=w7606, "Suffix"=w7629, "Interface in"=w7607) -> ("error out"=w7615:errorcluster, "Interface out"=w7621:refnum<class "Interface.lvclass">)  [unwired: 7 in]
            n3357 = call-dynamic "Write ObsType.vi"("error in (no error)"=w7615, "ObsType"=w7614, "Interface in"=w7621) -> ("error out"=w7616:errorcluster, "Interface out"=w7622:refnum<class "Interface.lvclass">)  [unwired: 7 in]
            n3358 = call-dynamic "Write Object.vi"("error in (no error)"=w7616, "Object"=w7613, "Interface in"=w7622) -> ("error out"=w7617:errorcluster, "Interface out"=w7623:refnum<class "Interface.lvclass">)  [unwired: 7 in]
            n3359 = call-dynamic "Write Comments.vi"("error in (no error)"=w7617, "Comments"=w7628, "Interface in"=w7623) -> ("error out"=w7609:errorcluster, "Interface out"=w7608:refnum<class "Interface.lvclass">)  [unwired: 7 in]
            n3360 = call-dynamic "Write Observer.vi"("error in (no error)"=w7609, "Observer"=w7612, "Interface in"=w7608) -> ("error out"=w7610:errorcluster, "Interface out"=w7611:refnum<class "Interface.lvclass">)  [unwired: 7 in]
            n3361 = call-dynamic "Write Interface.vi"("error in (no error)"=w7610, "Interface.lvclass"=w7611, "Channel in"=w7620) -> ("error out"=w7604:errorcluster, "Channel out"=w7605:refnum<class "Channel.lvclass">)  [unwired: 7 in]
            n3362 = disable-structure shown="Enabled" {
              disable-tunnel: w7605 -> [w7638 w7645]
              disable-tunnel: w7604 -> [w7637 w7644]
              disable-tunnel: [w7635 w7645] -> w7603
              disable-tunnel: [w7634 w7644] -> w7602
              frame Disabled {
                n3363 = call-dynamic "Read State Machine.vi"("error in (no error)"=w7637, "Device in"=w7638) -> ("error out"=w7643:errorcluster, "State Machine.lvclass"=w7641:refnum<class "State Machine.lvclass">, "Device out"=w7636:refnum<class "Channel.lvclass">)  [unwired: 7 in]
                n3364 = call "Next State.vi"("error in (no error)"=w7643, "New_State"=12, "State Machine in"=w7641) -> ("error out"=w7642:errorcluster, "State Machine out"=w7640:refnum<class "State Machine.lvclass">)  [unwired: 7 in]
                n3365 = call-dynamic "Write State Machine.vi"("error in (no error)"=w7642, "State Machine.lvclass"=w7640, "Device in"=w7636) -> ("error out"=w7634:errorcluster, "Device out"=w7635:refnum<class "Channel.lvclass">)  [unwired: 7 in]
              }
              frame Enabled {
              }
            }
            n3366 = call-dynamic "Write Channel.vi"("error in (no error)"=w7602, "Channel.lvclass"=w7603, "Acquisition in"=w7625) -> ("error out"=w7627:errorcluster, "Acquisition out"=w7626:refnum<class "Acquisition.lvclass">)  [unwired: 7 in]
            n3367 = call "Write AcquisitionB.vi"("error in (no error)"=w7627, "Acquisition.lvclass"=w7626, "S4ACS_GUI in"=w7624) -> ("error out"=w7630:errorcluster, "S4ACS_GUI out"=w7631:refnum<class "S4GUI.lvclass">)  [unwired: 7 in]
          }
          frame #2 {
            # "object"
            # "suffix"
            # "obsType"
            n3368 = call-dynamic "Read AcquisitionC.vi"("error in (no error)"=w7681, "S4ACS_GUI in"=w7682) -> ("error out"=w7674:errorcluster, "Acquisition.lvclass"=w7673:refnum<class "Acquisition.lvclass">, "S4ACS_GUI out"=w7668:refnum<class "S4GUI.lvclass">)  [unwired: 7 in]
            n3369 = call-dynamic "Read Channel.vi"("error in (no error)"=w7674, "Acquisition in"=w7673) -> ("error out"=w7648:errorcluster, "Channel.lvclass"=w7650:refnum<class "Channel.lvclass">, "Acquisition out"=w7667:refnum<class "Acquisition.lvclass">)  [unwired: 7 in]
            n3370 = local read "Filter3"() -> (w7651:u8)
            n3371 = call-dynamic "Write Filter.vi"("error in (no error)"=w7648, "Filter"=w7651, "Channel in"=w7650) -> ("error out"=w7647:errorcluster, "Channel out"=w7649:refnum<class "Channel.lvclass">)  [unwired: 7 in]
            n3372 = call-dynamic "Read Interface.vi"("error in (no error)"=w7647, "Channel in"=w7649) -> ("error out"=w7659:errorcluster, "Interface.lvclass"=w7660:refnum<class "Interface.lvclass">, "Channel out"=w7672:refnum<class "Channel.lvclass">)  [unwired: 7 in]
            n3373 = call-dynamic "Write Suffix.vi"("error in (no error)"=w7659, "Suffix"=w7678, "Interface in"=w7660) -> ("error out"=w7677:errorcluster, "Interface out"=w7671:refnum<class "Interface.lvclass">)  [unwired: 7 in]
            n3374 = call-dynamic "Write ObsType.vi"("error in (no error)"=w7677, "ObsType"=w7663, "Interface in"=w7671) -> ("error out"=w7676:errorcluster, "Interface out"=w7670:refnum<class "Interface.lvclass">)  [unwired: 7 in]
            n3375 = call-dynamic "Write Object.vi"("error in (no error)"=w7676, "Object"=w7662, "Interface in"=w7670) -> ("error out"=w7675:errorcluster, "Interface out"=w7669:refnum<class "Interface.lvclass">)  [unwired: 7 in]
            n3376 = call-dynamic "Write Comments.vi"("error in (no error)"=w7675, "Comments"=w7664, "Interface in"=w7669) -> ("error out"=w7656:errorcluster, "Interface out"=w7655:refnum<class "Interface.lvclass">)  [unwired: 7 in]
            n3377 = call-dynamic "Write Observer.vi"("error in (no error)"=w7656, "Observer"=w7661, "Interface in"=w7655) -> ("error out"=w7657:errorcluster, "Interface out"=w7658:refnum<class "Interface.lvclass">)  [unwired: 7 in]
            n3378 = call-dynamic "Write Interface.vi"("error in (no error)"=w7657, "Interface.lvclass"=w7658, "Channel in"=w7672) -> ("error out"=w7653:errorcluster, "Channel out"=w7654:refnum<class "Channel.lvclass">)  [unwired: 7 in]
            n3379 = disable-structure shown="Enabled" {
              disable-tunnel: w7654 -> [w7689 w7694]
              disable-tunnel: w7653 -> [w7688 w7693]
              disable-tunnel: [w7683 w7693] -> w7652
              disable-tunnel: [w7686 w7694] -> w7646
              frame Disabled {
                n3380 = call-dynamic "Read State Machine.vi"("error in (no error)"=w7688, "Device in"=w7689) -> ("error out"=w7692:errorcluster, "State Machine.lvclass"=w7685:refnum<class "State Machine.lvclass">, "Device out"=w7687:refnum<class "Channel.lvclass">)  [unwired: 7 in]
                n3381 = call "Next State.vi"("error in (no error)"=w7692, "New_State"=12, "State Machine in"=w7685) -> ("error out"=w7691:errorcluster, "State Machine out"=w7684:refnum<class "State Machine.lvclass">)  [unwired: 7 in]
                n3382 = call-dynamic "Write State Machine.vi"("error in (no error)"=w7691, "State Machine.lvclass"=w7684, "Device in"=w7687) -> ("error out"=w7683:errorcluster, "Device out"=w7686:refnum<class "Channel.lvclass">)  [unwired: 7 in]
              }
              frame Enabled {
              }
            }
            n3383 = call-dynamic "Write Channel.vi"("error in (no error)"=w7652, "Channel.lvclass"=w7646, "Acquisition in"=w7667) -> ("error out"=w7665:errorcluster, "Acquisition out"=w7666:refnum<class "Acquisition.lvclass">)  [unwired: 7 in]
            n3384 = call-dynamic "Write AcquisitionC.vi"("error in (no error)"=w7665, "Acquisition.lvclass"=w7666, "S4ACS_GUI in"=w7668) -> ("error out"=w7679:errorcluster, "S4ACS_GUI out"=w7680:refnum<class "S4GUI.lvclass">)  [unwired: 7 in]
          }
          frame #3 {
            # "object"
            # "suffix"
            # "obsType"
            n3385 = call-dynamic "Read AcquisitionD.vi"("error in (no error)"=w7730, "S4ACS_GUI in"=w7731) -> ("error out"=w7723:errorcluster, "Acquisition.lvclass"=w7722:refnum<class "Acquisition.lvclass">, "S4ACS_GUI out"=w7717:refnum<class "S4GUI.lvclass">)  [unwired: 7 in]
            n3386 = call-dynamic "Read Channel.vi"("error in (no error)"=w7723, "Acquisition in"=w7722) -> ("error out"=w7696:errorcluster, "Channel.lvclass"=w7698:refnum<class "Channel.lvclass">, "Acquisition out"=w7716:refnum<class "Acquisition.lvclass">)  [unwired: 7 in]
            n3387 = local read "Filter4"() -> (w7699:u8)
            n3388 = call-dynamic "Write Filter.vi"("error in (no error)"=w7696, "Filter"=w7699, "Channel in"=w7698) -> ("error out"=w7695:errorcluster, "Channel out"=w7697:refnum<class "Channel.lvclass">)  [unwired: 7 in]
            n3389 = call-dynamic "Read Interface.vi"("error in (no error)"=w7695, "Channel in"=w7697) -> ("error out"=w7708:errorcluster, "Interface.lvclass"=w7709:refnum<class "Interface.lvclass">, "Channel out"=w7721:refnum<class "Channel.lvclass">)  [unwired: 7 in]
            n3390 = call-dynamic "Write Suffix.vi"("error in (no error)"=w7708, "Suffix"=w7727, "Interface in"=w7709) -> ("error out"=w7726:errorcluster, "Interface out"=w7720:refnum<class "Interface.lvclass">)  [unwired: 7 in]
            n3391 = call-dynamic "Write ObsType.vi"("error in (no error)"=w7726, "ObsType"=w7712, "Interface in"=w7720) -> ("error out"=w7725:errorcluster, "Interface out"=w7719:refnum<class "Interface.lvclass">)  [unwired: 7 in]
            n3392 = call-dynamic "Write Object.vi"("error in (no error)"=w7725, "Object"=w7711, "Interface in"=w7719) -> ("error out"=w7724:errorcluster, "Interface out"=w7718:refnum<class "Interface.lvclass">)  [unwired: 7 in]
            n3393 = call-dynamic "Write Comments.vi"("error in (no error)"=w7724, "Comments"=w7713, "Interface in"=w7718) -> ("error out"=w7707:errorcluster, "Interface out"=w7706:refnum<class "Interface.lvclass">)  [unwired: 7 in]
            n3394 = call-dynamic "Write Observer.vi"("error in (no error)"=w7707, "Observer"=w7710, "Interface in"=w7706) -> ("error out"=w7705:errorcluster, "Interface out"=w7704:refnum<class "Interface.lvclass">)  [unwired: 7 in]
            n3395 = call-dynamic "Write Interface.vi"("error in (no error)"=w7705, "Interface.lvclass"=w7704, "Channel in"=w7721) -> ("error out"=w7701:errorcluster, "Channel out"=w7703:refnum<class "Channel.lvclass">)  [unwired: 7 in]
            n3396 = disable-structure shown="Enabled" {
              disable-tunnel: w7703 -> [w7738 w7743]
              disable-tunnel: [w7736 w7743] -> w7702
              disable-tunnel: w7701 -> [w7735 w7742]
              disable-tunnel: [w7734 w7742] -> w7700
              frame Disabled {
                n3397 = call-dynamic "Read State Machine.vi"("error in (no error)"=w7735, "Device in"=w7738) -> ("error out"=w7741:errorcluster, "State Machine.lvclass"=w7733:refnum<class "State Machine.lvclass">, "Device out"=w7737:refnum<class "Channel.lvclass">)  [unwired: 7 in]
                n3398 = call "Next State.vi"("error in (no error)"=w7741, "New_State"=12, "State Machine in"=w7733) -> ("error out"=w7740:errorcluster, "State Machine out"=w7732:refnum<class "State Machine.lvclass">)  [unwired: 7 in]
                n3399 = call-dynamic "Write State Machine.vi"("error in (no error)"=w7740, "State Machine.lvclass"=w7732, "Device in"=w7737) -> ("error out"=w7734:errorcluster, "Device out"=w7736:refnum<class "Channel.lvclass">)  [unwired: 7 in]
              }
              frame Enabled {
              }
            }
            n3400 = call-dynamic "Write Channel.vi"("error in (no error)"=w7700, "Channel.lvclass"=w7702, "Acquisition in"=w7716) -> ("error out"=w7714:errorcluster, "Acquisition out"=w7715:refnum<class "Acquisition.lvclass">)  [unwired: 7 in]
            n3401 = call-dynamic "Write AcquisitionD.vi"("error in (no error)"=w7714, "Acquisition.lvclass"=w7715, "S4ACS_GUI in"=w7717) -> ("error out"=w7728:errorcluster, "S4ACS_GUI out"=w7729:refnum<class "S4GUI.lvclass">)  [unwired: 7 in]
          }
        }
      }
      event "Start ch1": Value Change {
        n3402 = event-data() -> ()  [unwired: 1 in, 6 out]
        n3403 = call "Read Instrument.lvclass.vi"("error in (no error)"=w7753, "S4ACS_GUI in"=w7755) -> ("error out"=w7756:errorcluster, "Instrument.lvclass"=w7757:refnum<class "Instrument.lvclass">, "S4ACS_GUI out"=w7754:refnum<class "S4GUI.lvclass">)  [unwired: 7 in]
        n3404 = call-dynamic "Read mode.vi"("error in (no error)"=w7756, "Instrument in"=w7757) -> ("error out"=w7752:errorcluster, "mode"=w7751:bool)  [unwired: 7 in, 1 out]
        n3405 = call-dynamic "Read AcquisitionA.vi"("error in (no error)"=w7752, "S4ACS_GUI in"=w7754) -> ("error out"=w7769:errorcluster, "Acquisition.lvclass"=w7770:refnum<class "Acquisition.lvclass">, "S4ACS_GUI out"=w7772:refnum<class "S4GUI.lvclass">)  [unwired: 7 in]
        n3406 = call-dynamic "Read Acq_state.vi"("error in (no error)"=w7769, "Acquisition in"=w7770) -> ("error out"=w7766:errorcluster, "Acq_state"=w7768:u32, "Acquisition out"=w7765:refnum<class "Acquisition.lvclass">)  [unwired: 7 in]
        n3407 = Not Equal?(x=w7768, y=u32 400) -> (x != y?=w7771:bool)
        n3408 = case shown="True" w7771 {
          tunnel: w7772 -> [w7785 w7824]
          tunnel: [w7785 w7831] -> w7764
          tunnel: [w7780 w7830] -> w7748
          tunnel: w7766 -> [w7787 w7816]
          tunnel: w7765 -> [w7790 w7812]
          tunnel: [w7781 w7804] -> w7763
          tunnel: w7762 -> [_ w7849]
          tunnel: w7761 -> [_ w7848]
          tunnel: w7760 -> [_ w7847]
          tunnel: w7759 -> [_ w7846]
          tunnel: w7758 -> [_ w7841]
          tunnel: w7751 -> [_ w7829]
          tunnel: w7747 -> [_ w7807]
          tunnel: w7746 -> [_ w7810]
          tunnel: w7745 -> [_ w7809]
          tunnel: w7744 -> [_ w7808]
          frame False {
            n3409 = call-dynamic "Read Acq_prevstate.vi"("error in (no error)"=w7787, "Acquisition in"=w7790) -> ("error out"=w7786:errorcluster, "Acq_prevstate"=w7788:u32, "Acquisition out"=w7789:refnum<class "Acquisition.lvclass">)  [unwired: 7 in]
            n3410 = call-dynamic "Write Acq_state.vi"("error in (no error)"=w7786, "Acq_state"=w7788, "Acquisition in"=w7789) -> ("error out"=w7777:errorcluster, "Acquisition out"=w7779:refnum<class "Acquisition.lvclass">)  [unwired: 7 in]
            n3411 = call-dynamic "Read enabled.vi"("error in (no error)"=w7777, "Server in"=w7779) -> ("error out"=w7776:errorcluster, "enabled"=w7773:bool, "Server out"=w7778:refnum<class "Acquisition.lvclass">)  [unwired: 7 in]
            n3412 = call-dynamic "Read Channel.vi"("error in (no error)"=w7776, "Acquisition in"=w7778) -> ("error out"=w7774:errorcluster, "Channel.lvclass"=w7775:refnum<class "Channel.lvclass">, "Acquisition out"=w7784:refnum<class "Acquisition.lvclass">)  [unwired: 7 in]
            n3413 = case shown="True" w7773 {
              tunnel: w7775 -> [w7792 w7802]
              tunnel: [w7792 w7800] -> w7783
              tunnel: w7774 -> [w7791 w7797]
              tunnel: [w7791 w7795] -> w7782
              frame False {
              }
              frame True {
                n3414 = call-dynamic "Read State Machine.vi"("error in (no error)"=w7797, "Device in"=w7802) -> ("error out"=w7793:errorcluster, "State Machine.lvclass"=w7794:refnum<class "State Machine.lvclass">, "Device out"=w7801:refnum<class "Channel.lvclass">)  [unwired: 7 in]
                n3415 = call "Next State.vi"("error in (no error)"=w7793, "New_State"=96, "State Machine in"=w7794) -> ("error out"=w7796:errorcluster, "State Machine out"=w7799:refnum<class "State Machine.lvclass">)  [unwired: 7 in]
                n3416 = call-dynamic "Write State Machine.vi"("error in (no error)"=w7796, "State Machine.lvclass"=w7799, "Device in"=w7801) -> ("error out"=w7795:errorcluster, "Device out"=w7800:refnum<class "Channel.lvclass">)  [unwired: 7 in]
              }
            }
            n3417 = call-dynamic "Write Channel.vi"("error in (no error)"=w7782, "Channel.lvclass"=w7783, "Acquisition in"=w7784) -> ("error out"=w7780:errorcluster, "Acquisition out"=w7781:refnum<class "Acquisition.lvclass">)  [unwired: 7 in]
          }
          frame True {
            # "vide S4GUI:\nHandleObservationAsync.vi"
            # "object"
            # "suffix"
            # "obsType"
            n3418 = call "Read Instrument.lvclass.vi"("S4ACS_GUI in"=w7824) -> ("error out"=w7826:errorcluster, "Instrument.lvclass"=w7828:refnum<class "Instrument.lvclass">, "S4ACS_GUI out"=w7814:refnum<class "S4GUI.lvclass">)  [unwired: 8 in]
            n3419 = call "Read WPROT.vi"("error in (no error)"=w7826, "Instrument in"=w7828) -> ("error out"=w7825:errorcluster, "Opt_Selector.lvclass"=w7827:refnum<class "Opt_Selector.lvclass">)  [unwired: 7 in, 1 out]
            n3420 = call-dynamic "Read sequencia.vi"("error in (no error)"=w7825, "Opt_Selector in"=w7827) -> ("sequencia"=w7823:u16)  [unwired: 7 in, 2 out]
            n3421 = case shown="\"FOCUS\"" w7807 {
              tunnel: [u32 1 ("#cycles ch1") "#cycles ch1"] -> w7832
              tunnel: w7829 -> [_ w7880]
              tunnel: w7823 -> [_ w7879]
              tunnel: [u32 1 w7878] -> w7822
              frame "FOCUS" {
                # "Para sequência de foco, #cycles=1 e #seqs=1."
              }
              frame Default {
                n3422 = case shown="True" w7880 {
                  tunnel: [0 w7884] -> w7878
                  tunnel: w7879 -> [_ w7883]
                  frame False {
                    # "OV 20230424: \n#SEQ agora armazena as\nposições da lâmina utilizadas.\nNa fotometria, #SEQ=0"
                    # "fotometria:"
                  }
                  frame True {
                    # "OV 20230424: \n#SEQ agora armazena as\nposições da lâmina utilizadas.\nNa polarimetria, #SEQ=WPROT.sequencia"
                    # "polarimetria:"
                    n3423 = To Unsigned Long Integer(number=w7883) -> (unsigned 32bit integer=w7884:u32)
                  }
                }
              }
            }
            n3424 = case shown="\"FOCUS\"" w7807 {
              tunnel: [u32 271 ("Obs_state") u32 251 ("Obs_state")] -> w7815
              tunnel: w7816 -> [w7888 w7899]
              tunnel: [w7887 w7899] -> w7811
              tunnel: w7810 -> [w7895 _]
              tunnel: w7809 -> [w7894 _]
              tunnel: w7808 -> [w7893 _]
              tunnel: w7814 -> [w7886 w7898]
              tunnel: [w7885 w7898] -> w7813
              frame "FOCUS" {
                n3425 = call-dynamic "Read TelFocus.lvclass.vi"("error in (no error)"=w7888, "S4GUI in"=w7886) -> ("error out"=w7890:errorcluster, "TelFocus.lvclass"=w7892:refnum<class "TelFocus.lvclass">, "S4GUI out"=w7896:refnum<class "S4GUI.lvclass">)  [unwired: 7 in]
                n3426 = call-dynamic "LoadParam.vi"("#steps"=w7893, "error in (no error)"=w7890, "step"=w7894, "init"=w7895, "TelFocus in"=w7892) -> ("error out"=w7889:errorcluster, "TelFocus out"=w7891:refnum<class "TelFocus.lvclass">)  [unwired: 5 in]
                n3427 = call-dynamic "Write TelFocus.lvclass.vi"("error in (no error)"=w7889, "TelFocus.lvclass"=w7891, "S4GUI in"=w7896) -> ("error out"=w7887:errorcluster, "S4GUI out"=w7885:refnum<class "S4GUI.lvclass">)  [unwired: 7 in]
              }
              frame Default {
              }
            }
            n3428 = property on="Start ch1" class="Bool"(error in=w7816, "DisabledEnum"=T12."Disabled and Grayed Out" ("Disabled")) -> ()  [unwired: 1 in, 2 out]
            n3429 = call-dynamic "Write Acq_state.vi"("error in (no error)"=w7811, "Acq_state"=w7815, "Acquisition in"=w7812) -> ("error out"=w7850:errorcluster, "Acquisition out"=w7851:refnum<class "Acquisition.lvclass">)  [unwired: 7 in]
